vi "Auto Runner.vi"   [LabVIEW 2019]
doc: "This VI starts when autonomous period begins, and will automatically be terminated when it ends. You can carry out timed or sensor driven operations directly to I/O or to subsystems without needing to return to the caller."
uses:
  2020 Robot/Framework/Robot Global Data.vi
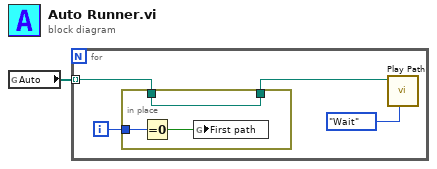
[diagram p0: block diagram]
diagram:
  n1 = global read "Robot Global Data.vi" "Auto"() -> (w1:path[])
  n2 = for {
    tunnel: w1 -> [w2] mode=indexing
    i -> [w4]
    n3 = in-place {
      in-place-border: w4 -> [w8]
      in-place-border: [w6] -> w3
      in-place-border: w2 -> [w6]
      n4 = Equal To 0?(x=w8) -> (x = 0?=w7:bool)
      n5 = global write "Robot Global Data.vi" "First path"(w7) -> ()
    }
    n6 = call "Play Path.vi"("Synchronication"=enum16{"Start", "Wait"}."Wait", "Path"=w3) -> ()  [unwired: 9 in, 1 out]
  }
